vi "Read Encoders.vi"(8 "Reset?":bool) -> (3 "Encoders":T1)   [LabVIEW 2015]
uses:
  Encoder Packet.ctl
  Single Encoder Data.ctl
  <vilib>/Rock Robotics/Network Tables/NT Read Number.vi
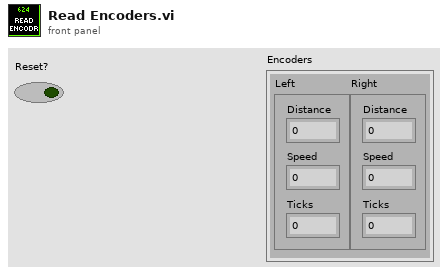
[diagram p1: front panel]
types:
  T1 = typedef "Encoder Packet.ctl" = cluster{"Left":T2, "Right":T2}
  T2 = typedef "Single Encoder Data.ctl" = cluster{"Distance":dbl, "Speed":dbl, "Ticks":dbl}
  T3 = typedef "WPI_EncoderDevRef.ctl" = cluster{"DevStatus":errorcluster, "EncoderIndex":T4, "CounterIndex":T5, "DistancePerCount":dbl, "Decoding Type":T6}
  T4 = typedef "FPGA_EncoderIdx.ctl" = enum8{"Enc 0", "Enc 1", "Enc 2", "Enc 3", "Enc 4", "Enc 5", "Enc 6", "Enc 7", "Invalid"}
  T5 = typedef "FPGA_CounterCtrSystemIndex.ctl" = enum8{"Ctr 0", "Ctr 1", "Ctr 2", "Ctr 3", "Ctr 4", "Ctr 5", "Ctr 6", "Ctr 7", "Invalid"}
  T6 = typedef "WPI_EncoderType.ctl" = enum16{"1x", "2x", "4x"}
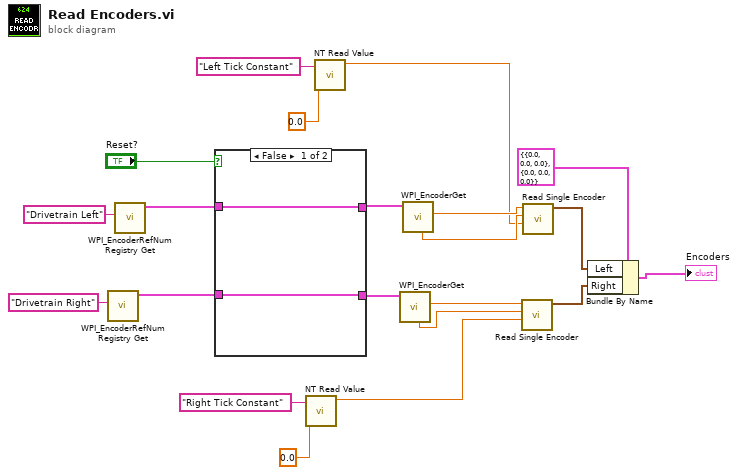
[diagram p0: block diagram]
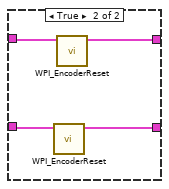
[diagram p2: hidden frame]
diagram:
  n1 = call <vilib>:"WPI_EncoderRefNum Registry Get.vi"("refnum name"="Drivetrain Right") -> ("EncoderDevRef"=w17:T3)  [unwired: 9 in, 1 out]
  n2 = call <vilib>:"WPI_EncoderRefNum Registry Get.vi"("refnum name"="Drivetrain Left") -> ("EncoderDevRef"=w18:T3)  [unwired: 9 in, 1 out]
  n3 = case shown="False" "Reset?" {
    tunnel: w18 -> [w23 w27]
    tunnel: w17 -> [w22 w25]
    tunnel: [w23 w26] -> w11
    tunnel: [w22 w24] -> w12
    frame False {
    }
    frame True {
      n4 = call <vilib>:"WPI_EncoderReset.vi"("EncoderDevRef"=w25) -> ("EncoderDevRef"=w24:T3)  [unwired: 9 in, 1 out]
      n5 = call <vilib>:"WPI_EncoderReset.vi"("EncoderDevRef"=w27) -> ("EncoderDevRef"=w26:T3)  [unwired: 9 in, 1 out]
    }
  }
  n6 = call-poly <vilib>:"NT Read Value.vi"("Default Value"=0.0, "Name"="Right Tick Constant") -> ("Numeric"=w9:dbl)  [unwired: 8 in, 1 out]
  n7 = call-poly <vilib>:"NT Read Value.vi"("Default Value"=0.0, "Name"="Left Tick Constant") -> ("Numeric"=w5:dbl)  [unwired: 8 in, 1 out]
  n8 = call <vilib>:"WPI_EncoderGet.vi"("EncoderDevRef"=w12) -> ("Distance"=w8:dbl, "Rate"=w10:dbl)  [unwired: 5 in, 4 out]
  n9 = call <vilib>:"WPI_EncoderGet.vi"("EncoderDevRef"=w11) -> ("Distance"=w7:dbl, "Rate"=w6:dbl)  [unwired: 5 in, 4 out]
  n10 = call "Read Single Encoder.vi"("TC"=w9, "Rate"=w10, "Distance"=w8) -> ("Single Encoder Data 2"=w3:T2)  [unwired: 8 in]
  n11 = call "Read Single Encoder.vi"("TC"=w5, "Rate"=w6, "Distance"=w7) -> ("Single Encoder Data 2"=w2:T2)  [unwired: 8 in]
  n12 = Bundle By Name(cluster=T1 {"Left"={"Distance"=0.0, "Speed"=0.0, "Ticks"=0.0}, "Right"={"Distance"=0.0, "Speed"=0.0, "Ticks"=0.0}} ("Encoders"), "Left"=w2, "Right"=w3) -> (→"Encoders":T1)
